vi "arreglo3.vi"() -> ()   [LabVIEW 2011]
uses:
  arreglo3.ctl
  <vilib>/express/express arith-compare/Formula/XNode/ExpressFormulaBlockNode.xnode
panel:
  out "Array 2":string[](array[string])
  out "Array":dbl[](array[numeric])
  # "En el arreglo 1 ingresar 5 numeros enteros y luego en el arreglo 2\nescribir si es par o impar cada uno de los numeros"
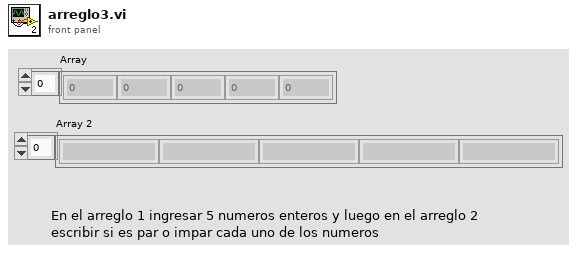
[diagram p1: front panel]
types:
  T1 = typedef "arreglo3.ctl" = enum16{"iniciar arreglos", "rellenar arreglo1", "encontrarPareImpares", "final"}
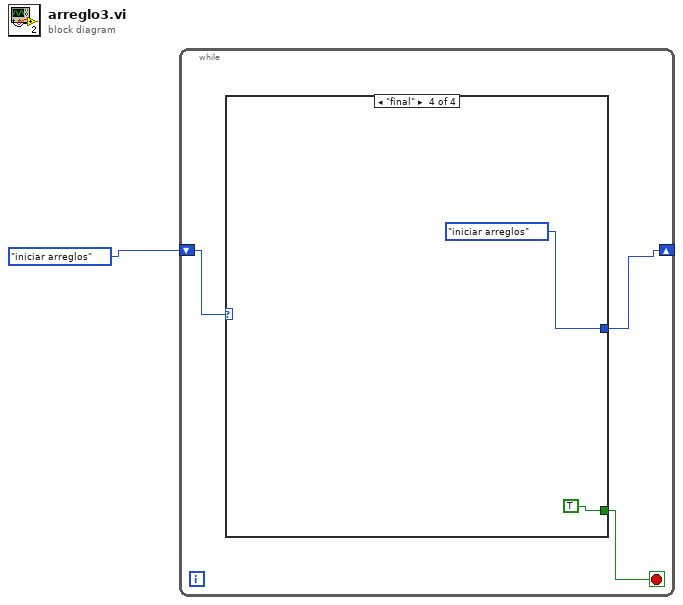
[diagram p0: block diagram]
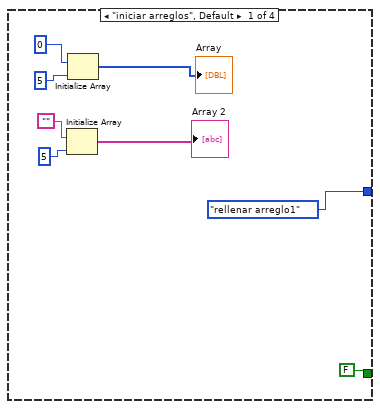
[diagram p2: hidden frame]
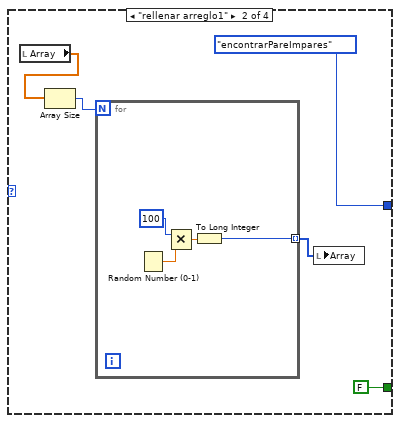
[diagram p3: hidden frame]
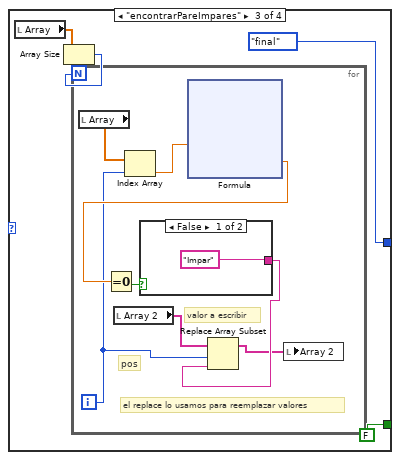
[diagram p4: hidden frame]
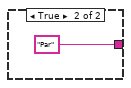
[diagram p5: hidden frame]
diagram:
  n1 = while {
    shift-right: [w3] -> _
    shift-left: arreglo3."iniciar arreglos" -> [w4]
    stop <- w2 stop-if-true
    n2 = case shown="\"final\"" w4 {
      tunnel: [arreglo3."rellenar arreglo1" arreglo3."encontrarPareImpares" arreglo3."final" arreglo3."iniciar arreglos"] -> w3
      tunnel: [FALSE FALSE FALSE TRUE] -> w2
      frame "iniciar arreglos", Default {
        n3 = Initialize Array "Initialize Array"("", 5) -> (→"Array 2":string[])
        n4 = Initialize Array "Initialize Array"(0, 5) -> (→"Array":i32[])
      }
      frame "rellenar arreglo1" {
        n5 = local read "Array"() -> (w15:dbl[])
        n6 = Array Size(array=w15) -> (size(s)=w16:i32)
        n7 = for {
          N: w16 -> [_]
          tunnel: [w18] -> w14 mode=indexing
          n8 = Random Number (0-1)() -> (number: 0 to 1=w21:dbl)
          n9 = Multiply(x=100, y=w21) -> (x*y=w19:dbl)
          n10 = To Long Integer(number=w19) -> (32bit integer=w18:i32)
        }
        n11 = local write "Array"(w14) -> ()
      }
      frame "encontrarPareImpares" {
        n12 = local read "Array"() -> (w24:dbl[])
        n13 = Array Size(array=w24) -> (size(s)=w25:i32)
        n14 = for {
          N: w25 -> [_]
          i -> [w28]
          # "el replace lo usamos para reemplazar valores"
          # "valor a escribir"
          # "pos"
          n15 = local read "Array"() -> (w33:dbl[])
          n16 = local read "Array 2"() -> (w29:string[])
          n17 = Index Array "Index Array"(array=w33, index=w28) -> (element=w30:dbl)
          n18 = xnode "Formula"("X1"=w30) -> ("Result"=w31:dbl)  [unwired: 1 in, 1 out]
          n19 = Equal To 0?(x=w31) -> (x = 0?=w32:bool)
          n20 = case shown="False" w32 {
            tunnel: ["Impar" "Par"] -> w27
            frame False {
            }
            frame True {
            }
          }
          n21 = Replace Array Subset "Replace Array Subset"(array=w29, new element=w27, index=w28) -> (w26:string[])
          n22 = local write "Array 2"(w26) -> ()
        }
      }
      frame "final" {
      }
    }
  }
